vi "AlliGator Save Hot Pixel Mask Image.vi"(8 "error in (no error)":errorcluster, 9 "Saved Image File Format":T2, 10 "File Path in":path, 11 "Image Refnum in":T1) -> (0 "Error Out":errorcluster, 2 "File Path out":path)   [LabVIEW 2021, in "AlliGator Files.lvlib"]
doc: "Saves image as 8-bit binary Mask Image."
uses:
  AlliGator Files.lvlib
  Image/Image Save File Format.ctl
  <vilib>/vision/Image Controls.llb/IMAQ Image.ctl
  Image/Image.lvlib
panel:
  # "see the AlliGator License on the block diagram (Ctrl+E or Window:Show Block Diagram)"
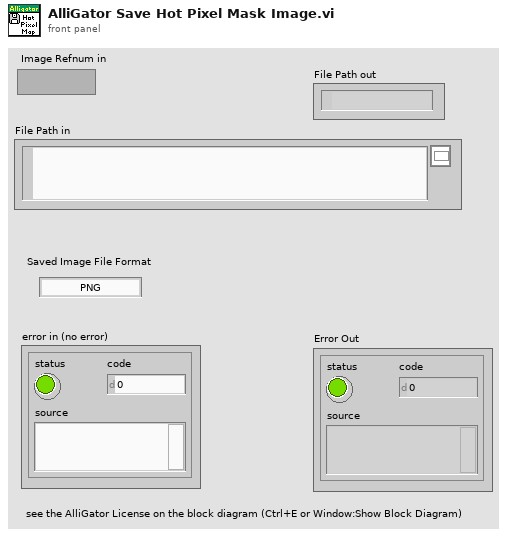
[diagram p1: front panel]
types:
  T1 = typedef "IMAQ Image.ctl" = refnum<image>
  T2 = typedef "Image.lvlib/Image Save File Format.ctl" = enum16{"PNG", "JPEG", "BMP"}
  T3 = typedef "Image Type" = u32
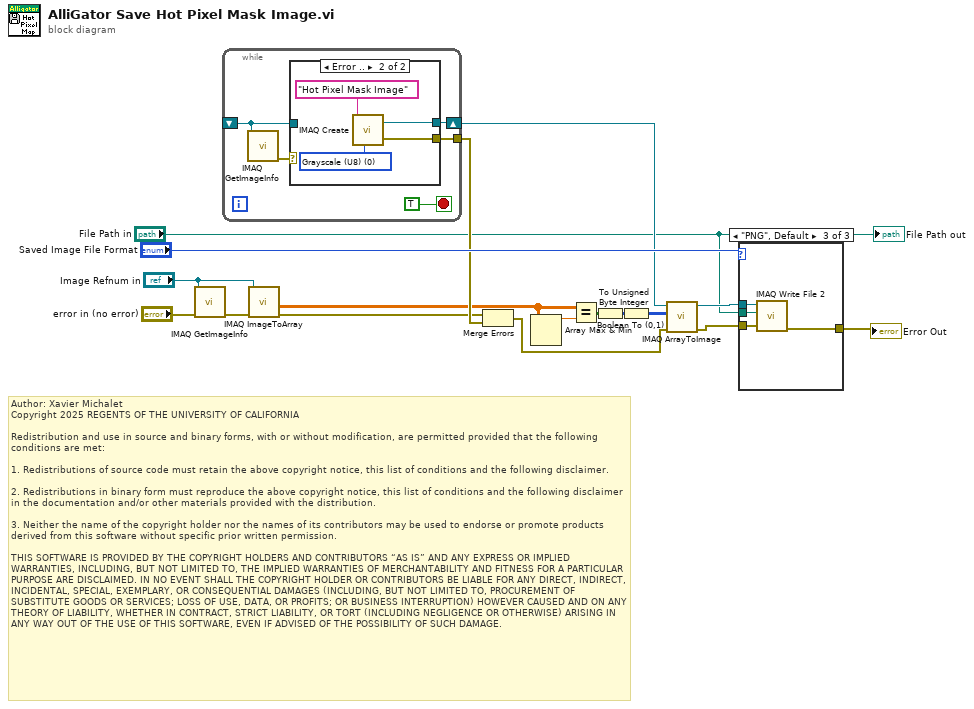
[diagram p0: block diagram]
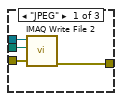
[diagram p2: hidden frame]
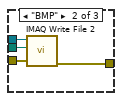
[diagram p3: hidden frame]
diagram:
  # "Author: Xavier Michalet\nCopyright 2025 REGENTS OF THE UNIVERSITY OF CALIFORNIA\n\nRedistribution and use in source and binary forms, with or without modification, are permitted provided that the following conditions are met:\n\n1. Redistributions of source code must retain the above copyright notice, this list of conditions and the following disclaimer.\n\n2. Redistributions in binary form must reproduce the above copyright notice, this list of conditions and the following disclaimer in the documentation and/or other materials provided with the distribution.\n\n3. Neither the name of the copyright holder nor the names of its contributors may be used to endorse or promote products derived from this software without specific prior written permission.\n\nTHIS SOFTWARE IS PROVIDED BY THE COPYRIGHT HOLDERS AND CONTRIBUTORS “AS IS” AND ANY EXPRESS OR IMPLIED WARRANTIES, INCLUDING, BUT NOT LIMITED TO, THE IMPLIED WARRANTIES OF MERCHANTABILITY AND FITNESS FOR A PARTICULAR PURPOSE ARE DISCLAIMED. IN NO EVENT SHALL THE COPYRIGHT HOLDER OR CONTRIBUTORS BE LIABLE FOR ANY DIRECT, INDIRECT, INCIDENTAL, SPECIAL, EXEMPLARY, OR CONSEQUENTIAL DAMAGES (INCLUDING, BUT NOT LIMITED TO, PROCUREMENT OF SUBSTITUTE GOODS OR SERVICES; LOSS OF USE, DATA, OR PROFITS; OR BUSINESS INTERRUPTION) HOWEVER CAUSED AND ON ANY THEORY OF LIABILITY, WHETHER IN CONTRACT, STRICT LIABILITY, OR TORT (INCLUDING NEGLIGENCE OR OTHERWISE) ARISING IN ANY WAY OUT OF THE USE OF THIS SOFTWARE, EVEN IF ADVISED OF THE POSSIBILITY OF SUCH DAMAGE."
  n1 = call "IMAQ GetImageInfo"("error in (no error)"="error in (no error)", "Image"="Image Refnum in") -> ("error out"=w15:errorcluster)  [unwired: 2 in, 7 out]
  n2 = while {
    shift-right: [w21] -> w9
    shift-left: _ -> [w20]
    tunnel: [w19] -> w12
    stop <- TRUE stop-if-true
    n3 = call "IMAQ GetImageInfo"("Image"=w20) -> ("error out"=w18:errorcluster)  [unwired: 3 in, 7 out]
    n4 = case shown="Error .." w18 {
      selector: w18 -> [w23 _]
      tunnel: [w24 w27] -> w21
      tunnel: w20 -> [w24 _]
      tunnel: [w23 w26] -> w19
      frame No Error {
      }
      frame Error {
        w25 = T3 0 items=["Grayscale (U8)", "Grayscale (I16)", "Grayscale (SGL)", "Complex (CSG)", "RGB (U32)", "HSL (U32)", "RGB (U64)", "Grayscale (U16)"] ("Image Type")
        n5 = call "IMAQ Create"("Image Name"="Hot Pixel Mask Image", "Image Type"=w25) -> ("New Image"=w27:T1, "error out"=w26:errorcluster)  [unwired: 3 in]
      }
    }
  }
  n6 = call "IMAQ ImageToArray"("error in (no error)"=w15, "Image"="Image Refnum in") -> ("Image Pixels (Float)"=w4:sgl[][], "error out"=w10:errorcluster)  [unwired: 2 in, 3 out]
  n7 = Merge Errors(w10, w12) -> (w11:errorcluster)
  n8 = Array Max & Min(array=w4) -> (max value=w5:sgl)  [unwired: 3 out]
  n9 = Equal?(x=w4, y=w5) -> (x = y?=w3:bool[][])
  n10 = Boolean To (0,1)(Boolean=w3) -> (0, 1=w2:i16[][])
  n11 = To Unsigned Byte Integer(number=w2) -> (unsigned 8bit integer=w1:u8[][])
  n12 = call "IMAQ ArrayToImage"("error in (no error)"=w11, "Image Pixels (U8)"=w1, "Image"=w9) -> ("error out"=w8:errorcluster, "Image Out"=w7:T1)  [unwired: 7 in]
  n13 = case shown="\"PNG\", Default" "Saved Image File Format" {
    tunnel: w8 -> [w32 w36 w40]
    tunnel: w7 -> [w31 w35 w39]
    tunnel: [w30 w34 w38] -> w16
    tunnel: "File Path in" -> [w29 w33 w37]
    frame "JPEG" {
      n14 = call-poly "IMAQ Write File 2"("error in (no error)"=w32, "File Path"=w29, "Image"=w31) -> ("error out"=w30:errorcluster)  [unwired: 7 in, 1 out]
    }
    frame "BMP" {
      n15 = call-poly "IMAQ Write File 2"("error in (no error)"=w36, "File Path"=w33, "Image"=w35) -> ("error out"=w34:errorcluster)  [unwired: 7 in, 1 out]
    }
    frame "PNG", Default {
      n16 = call-poly "IMAQ Write File 2"("error in (no error)"=w40, "File Path"=w37, "Image"=w39) -> ("error out"=w38:errorcluster)  [unwired: 7 in, 1 out]
    }
  }
  "Error Out" <- w16
  "File Path out" <- "File Path in"
